vi "GetData.vi"() -> (3 "Keys Pressed":T2(array[ring]))   [LabVIEW 2017]
doc: "This VI shows how to use the Input Device Control VIs. It displays keyboard and mouse activity while the VI is running. The Input Device Control VIs can also be used to display joystick information."
uses:
  <vilib>/Utility/inputDevices.llb/keyboardAcquire.vi
  <vilib>/Utility/inputDevices.llb/closeKeyboard.vi
panel:
  out "Stop_mercury":bool
  out "error out":errorcluster
  out "temp_mercury":dbl
  out "Numeric":i16
  out "element":T1(ring)
  # "Overview: Demonstrates the use of the Input Device Control VIs to monitor mouse and keyboard actions.\nRequirements: Windows or Linux\nInstructions:\n1. Run the VI.\n2. Observe the values of the indicators update as you press keyboard keys, change the mouse position, and click mouse buttons.\n3. Click Stop to stop the VI."
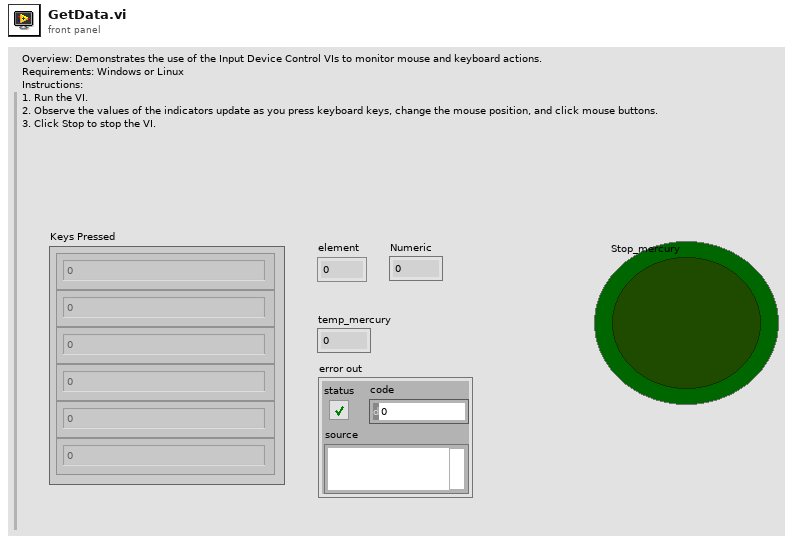
[diagram p1: front panel]
types:
  T1 = enum16{"0", "1", "2", "3", "4", "5", "6", "7", "8", "9", "A", "B", "C", "D", "E", "F", "G", "H", "I", "J", "K", "L", "M", "N", "O", "P", "Q", "R", "S", "T", "U", "V", "W", "X", "Y", "Z", "F1", "F2", "F3", "F4", "F5", "F6", "F7", "F8", "F9", "F10", "F11", "F12", "F13", "F14", "F15", "ADD", "BACK", "BACKSLASH", "CAPITAL", "COMMA", "DECIMAL", "DELETE", "DIVIDE", "DOWN", "END", "EQUALS", "ESCAPE", "GRAVE (`)", "HOME", "INSERT", "LBRACKET", "LCONTROL", "LEFT", "L ALT", "LSHIFT", "LWIN", "MINUS", "MULTIPLY", "NEXT", "NUMLOCK", "NUMPAD_0", "NUMPAD_1", "NUMPAD_2", "NUMPAD_3", "NUMPAD_4", "NUMPAD_5", "NUMPAD_6", "NUMPAD_7", "NUMPAD_8", "NUMPAD_9", "PAUSE", "PERIOD", "PRIOR (PG UP)", "RBRACKET", "RCONTROL", "RETURN", "RIGHT", "R ALT", "RSHIFT", "RWIN", "SCROLL", "SEMICOLON", "SLASH", "SPACE", "SUBTRACT", "TAB", "UP", "ENTER (num pad)", "' (quote)"}
  T2 = enum16{"0", "1", "2", "3", "4", "5", "6", "7", "8", "9", "A", "B", "C", "D", "E", "F", "G", "H", "I", "J", "K", "L", "M", "N", "O", "P", "Q", "R", "S", "T", "U", "V", "W", "X", "Y", "Z", "F1", "F2", "F3", "F4", "F5", "F6", "F7", "F8", "F9", "F10", "F11", "F12", "F13", "F14", "F15", "ADD", "BACK", "BACKSLASH", "CAPITAL", "COMMA", "DECIMAL", "DELETE", "DIVIDE", "DOWN", "END", "EQUALS", "ESCAPE", "GRAVE (`)", "HOME", "INSERT", "LBRACKET", "LCONTROL", "LEFT", "L ALT", "LSHIFT", "LWIN", "MINUS", "MULTIPLY", "NEXT", "NUMLOCK", "NUMPAD_0", "NUMPAD_1", "NUMPAD_2", "NUMPAD_3", "NUMPAD_4", "NUMPAD_5", "NUMPAD_6", "NUMPAD_7", "NUMPAD_8", "NUMPAD_9", "PAUSE", "PERIOD", "PRIOR (PG UP)", "RBRACKET", "RCONTROL", "RETURN", "RIGHT", "R ALT", "RSHIFT", "RWIN", "SCROLL", "SEMICOLON", "SLASH", "SPACE", "SUBTRACT", "TAB", "UP", "ENTER (num pad)", "' (quote)"}[]
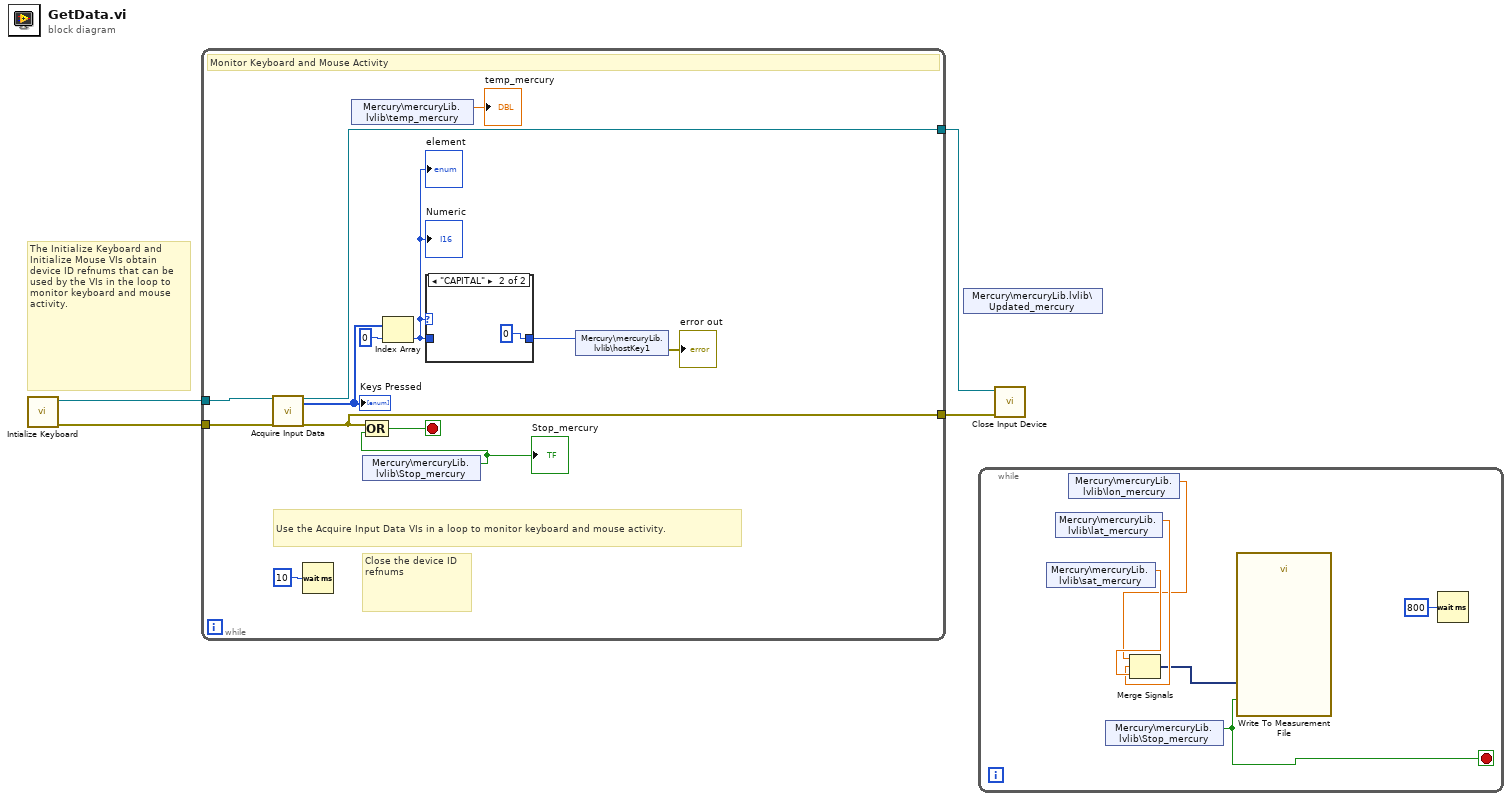
[diagram p0: block diagram]
diagram:
  # "The Initialize Keyboard and Initialize Mouse VIs obtain device ID refnums that can be used by the VIs in the loop to monitor keyboard and mouse activity."
  n1 = call <vilib>:"Intialize Keyboard.vi"() -> ("error out"=w3:errorcluster, "device ID"=w4:refnum<k1>)  [unwired: 1 in, 9 out]
  n2 = while {
    tunnel: [w12] -> w1
    tunnel: w3 -> [w17]
    tunnel: [w15] -> w2
    tunnel: w4 -> [w14]
    stop <- w13 stop-if-true
    # "Close the device ID refnums"
    # "Use the Acquire Input Data VIs in a loop to monitor keyboard and mouse activity."
    # "Monitor Keyboard and Mouse Activity"
    n3 = call-poly <vilib>:"Acquire Input Data.vi"("device ID"=w14, "error in (no error)"=w17) -> ("device ID"=w15:refnum<k1>, "keys pressed"=w10:T2, "error out"=w12:errorcluster)  [unwired: 15 out]
    "Keys Pressed" <- w10
    n4 = Wait (ms)(milliseconds to wait=u32 10) -> ()  [unwired: 1 out]
    n5 = shared-variable "Mercury\\mercuryLib.lvlib\\temp_mercury"() -> (→"temp_mercury":dbl)  [unwired: 1 in, 1 out]
    n6 = shared-variable "Mercury\\mercuryLib.lvlib\\Stop_mercury"() -> (w5:bool)  [unwired: 1 in, 1 out]
    "Stop_mercury" <- w5
    n7 = Compound Arithmetic op=OR(w12, w5) -> (w13:bool)
    n8 = Index Array(array=w10, index=0) -> (element=w6:T1)
    "element" <- w6
    "Numeric" <- w6
    n9 = case shown="\"CAPITAL\"" w6 {
      tunnel: [w18 0] -> w7
      tunnel: w6 -> [w18 _]
      frame "0", Default {
      }
      frame "CAPITAL" {
      }
    }
    n10 = shared-variable "Mercury\\mercuryLib.lvlib\\hostKey1"(w7) -> (error out=→"error out":errorcluster)  [unwired: 1 in]
  }
  n11 = shared-variable "Mercury\\mercuryLib.lvlib\\Updated_mercury"() -> ()  [unwired: 1 in, 2 out]
  n12 = while {
    stop <- w20 stop-if-true
    n13 = shared-variable "Mercury\\mercuryLib.lvlib\\sat_mercury"() -> (w25:dbl)  [unwired: 1 in, 1 out]
    n14 = shared-variable "Mercury\\mercuryLib.lvlib\\lat_mercury"() -> (w24:dbl)  [unwired: 1 in, 1 out]
    n15 = shared-variable "Mercury\\mercuryLib.lvlib\\lon_mercury"() -> (w23:dbl)  [unwired: 1 in, 1 out]
    n16 = shared-variable "Mercury\\mercuryLib.lvlib\\Stop_mercury"() -> (w20:bool)  [unwired: 1 in, 1 out]
    n17 = Merge Signals(w23, w24, w25) -> (w22:dynamicdata)
    n18 = call "Write To Measurement File"("Signals"=w22, "Flush? (T)"=w20) -> ()  [unwired: 15 in, 3 out]
    n19 = Wait (ms)(milliseconds to wait=u32 800) -> ()  [unwired: 1 out]
  }
  n20 = call-poly <vilib>:"Close Input Device.vi"("error in (no error)"=w1, "device ID"=w2) -> ()  [unwired: 9 out]
